vi "АЛУ(одноразрядное).vi"(2 "c":T1, 3 "c-1":bool, 4 "b":bool, 5 "a":bool) -> (0 "s1":bool, 1 "r":bool)   [LabVIEW 2013]
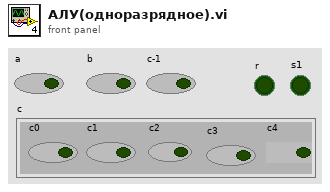
[diagram p1: front panel]
types:
  T1 = cluster{"c0":bool, "c1":bool, "c2":bool, "c3":bool, "c4":bool}
  T2 = cluster{"c1":bool, "c2":bool, "c3":bool, "c4":bool}
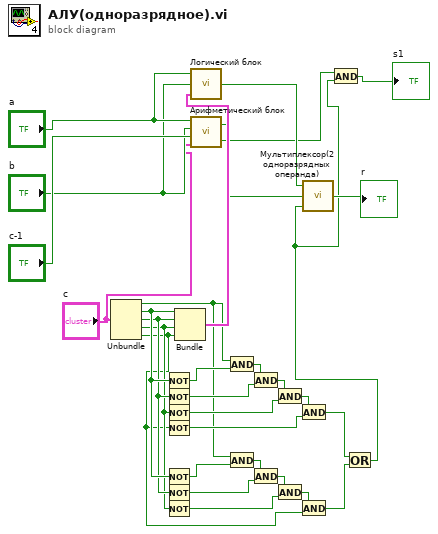
[diagram p0: block diagram]
diagram:
  n1 = Unbundle("c") -> ("c0"=w10:bool, "c1"=w9:bool, "c2"=w8:bool, "c3"=w7:bool, "c4"=w6:bool)
  n2 = Not(x=w9) -> (.not. x?=w23:bool)
  n3 = Not(x=w8) -> (.not. x?=w22:bool)
  n4 = Not(x=w7) -> (.not. x?=w21:bool)
  n5 = Not(x=w6) -> (.not. x?=w20:bool)
  n6 = Not(x=w9) -> (.not. x?=w16:bool)
  n7 = Not(x=w8) -> (.not. x?=w15:bool)
  n8 = Not(x=w7) -> (.not. x?=w14:bool)
  n9 = Bundle("c1"=w9, "c2"=w8, "c3"=w7, "c4"=w6) -> (w28:T2)  [unwired: 1 in]
  n10 = call "Логический блок.vi"("c"=w28, "b"="b", "a"="a") -> ("r"=w26:bool)
  n11 = call "Арифметический блок.vi"("c"="c", "c-1"="c-1", "b"="b", "a"="a") -> ("c"=w2:bool, "s"=w25:bool)
  n12 = And(x=w10, y=w23) -> (x .and. y?=w17:bool)
  n13 = And(x=w10, y=w16) -> (x .and. y?=w11:bool)
  n14 = And(x=w17, y=w22) -> (x .and. y?=w18:bool)
  n15 = And(x=w11, y=w15) -> (x .and. y?=w12:bool)
  n16 = And(x=w18, y=w21) -> (x .and. y?=w19:bool)
  n17 = And(x=w12, y=w14) -> (x .and. y?=w13:bool)
  n18 = And(x=w19, y=w20) -> (x .and. y?=w5:bool)
  n19 = And(x=w13, y=w6) -> (x .and. y?=w4:bool)
  n20 = Or(x=w5, y=w4) -> (x .or. y?=w1:bool)
  n21 = call "Мультиплексор(2 одноразрядных операнда).vi"("c"=w1, "y"=w25, "x"=w26) -> ("r"=→"r":bool)
  n22 = And(x=w2, y=w1) -> (x .and. y?=→"s1":bool)
